vi "Practica_Act02.vi"() -> ()   [LabVIEW 2020]
panel:
  in  "stop":bool
  out "Thermometer":dbl(slide) scale=0.0..80.0
  in  "Mustras":dbl(slide) scale=0.0..200.0
  in  "Tiempo de muestreo":dbl(slide) scale=0.0..10.0
  out "voltaje salida sensor":dbl
  in  "tiempo de espera del loop":dbl(slide) scale=0.0..1000.0
  out "Temperatura":dbl
  out "Waveform Chart":dynamicdata(graph)
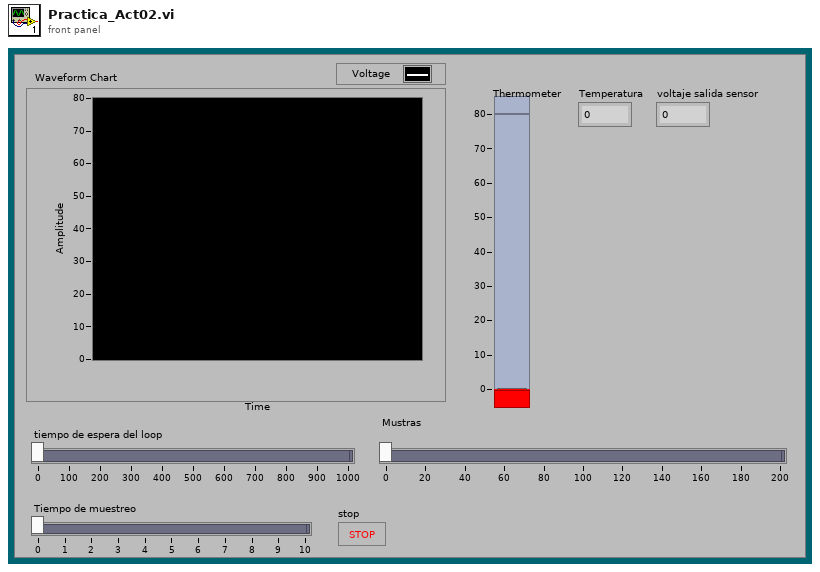
[diagram p1: front panel]
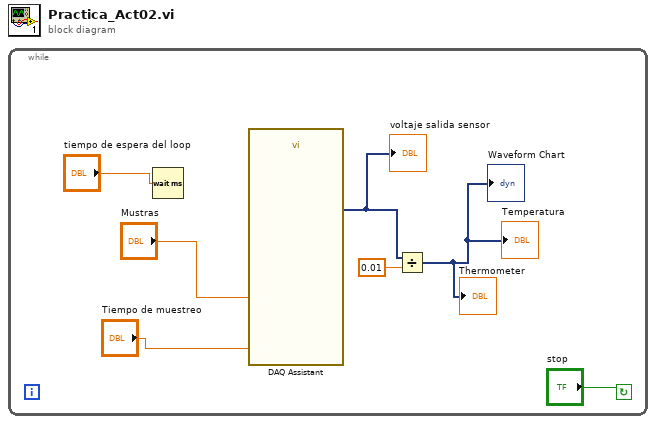
[diagram p0: block diagram]
diagram:
  n1 = while {
    stop <- "stop" continue-if-true
    n2 = Wait (ms)(milliseconds to wait="tiempo de espera del loop") -> ()  [unwired: 1 out]
    n3 = call "DAQ Assistant"("number of samples"="Mustras", "timeout (s)"="Tiempo de muestreo") -> ("data"=w6:dynamicdata)  [unwired: 15 in, 2 out]
    "voltaje salida sensor" <- w6
    n4 = Divide(x=w6, y=0.01) -> (x/y=→"Waveform Chart" →"Thermometer" →"Temperatura":dynamicdata)
  }
